vi "Untitled 2.vi"() -> ()   [LabVIEW 2015]
panel:
  in  "Sensor Position (degrees)":dbl
  in  "Goal Angle Degrees 0=straight ahead":dbl
  in  "Goal Detected":bool
  out "Finished?":bool
  out "Output":dbl
  in  "Yaw (degrees 0 = straight ahead gets larger clockwise)":dbl
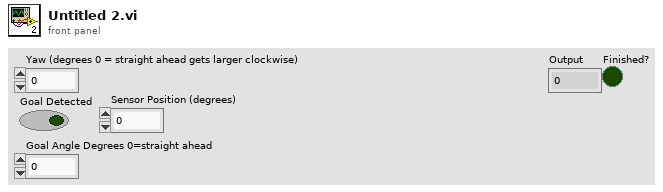
[diagram p1: front panel]
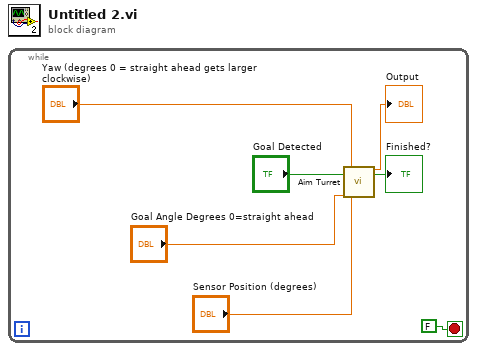
[diagram p0: block diagram]
diagram:
  n1 = while {
    stop <- FALSE stop-if-true
    n2 = call "Aim Turret.vi"("Goal Detected"="Goal Detected", "Goal Angle Degrees 0=straight ahead"="Goal Angle Degrees 0=straight ahead", "Yaw (degrees 0 = straight ahead gets larger clockwise)"="Yaw (degrees 0 = straight ahead gets larger clockwise)", "Sensor Position (degrees)"="Sensor Position (degrees)") -> ("Output"=→"Output":dbl, "Finished?"=→"Finished?":bool)  [unwired: 14 in]
  }
